vi "Write Wait Time.vi"(8 "error in (no error)":errorcluster, 10 "Wait Time":dbl, 11 "Wait in":refnum<class "Wait.lvclass">) -> (0 "error out":errorcluster, 3 "Wait out":refnum<class "Wait.lvclass">)   [LabVIEW 2015, in "Wait.lvclass"]
uses:
  Wait.lvclass
  Wait.lvclass/Wait.ctl
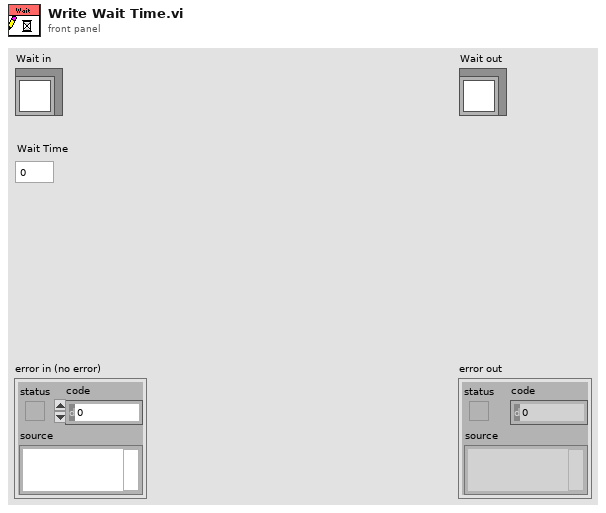
[diagram p1: front panel]
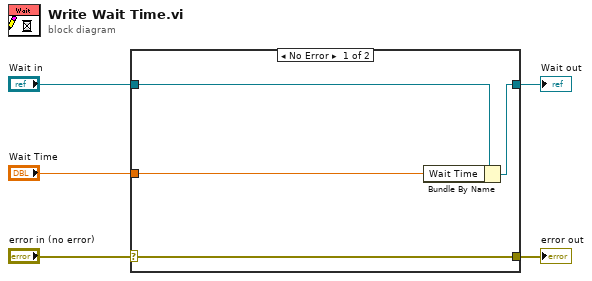
[diagram p0: block diagram]
diagram:
  n1 = case shown="No Error" "error in (no error)" {
    selector: "error in (no error)" -> [w9 w10]
    tunnel: [w9 w10] -> w4
    tunnel: [w7 w11] -> w2
    tunnel: "Wait in" -> [w8 w11]
    tunnel: "Wait Time" -> [w6 _]
    frame No Error {
      n2 = Bundle By Name(cluster=w8, "Wait Time"=w6) -> (w7:refnum<class "Wait.lvclass">)
    }
    frame Error {
    }
  }
  "error out" <- w4
  "Wait out" <- w2
